vi "Requests.vi"(8 "error in (no error)":errorcluster, 9 "write enable":bool=TRUE, 11 "ICPCON ET-7051 in":refnum<class "ICPCON ET-7051.lvclass">) -> (0 "error out":errorcluster, 3 "ICPCON ET-7051 out":refnum<class "ICPCON ET-7051.lvclass">)   [LabVIEW 2019, in "ICPCON ET-7051.lvclass"]
uses:
  ICPCON ET-7051.lvclass
  D:/my_projects/projects/Algorithms/Labview/19/Modbus/MB_TCP2/MB_TCP.lvclass
  MB_TCP.lvclass/MB_TCP.ctl
  NI_modbus_upd/Ctl/Unit_ID.ctl
  NI_modbus_upd/TCP/TCP.lvclass/TCP.ctl
  NI_modbus_upd/Master Function Definition/Responses/Read Discrete Inputs Response.vi
  NI_modbus_upd/Master network read write.vi
  NI_modbus_upd/Master Function Definition/Requests/Read Discrete Inputs Request.vi
  NI_modbus_upd/Utility/Bytes to Bits1.vi
  NI_modbus_upd/Function code mismatch error1.vi
  NI_modbus_upd/Error Generator1.vi
  NI_modbus_upd/Read ADU Packet Master.vi
  NI_modbus_upd/Write ADU Packet Master.vi
  NI_modbus_upd/Modbus Data Unit (PDU)/Construct PDU1.vi
  NI_modbus_upd/Modbus Data Unit (PDU)/Unflatten to PDU1.vi
  NI_modbus_upd/TCP/Protocol Read.vi
  NI_modbus_upd/TCP/Protocol Write.vi
  <vilib>/Utility/error.llb/Clear Errors.vi
  NI_modbus_upd/Modbus Data Unit (PDU)/Deconstruct PDU1.vi
  NI_modbus_upd/TCP/TCP.lvclass
  ICPCON Registers/ICPCON Registers.lvlib
  MB_TCP.lvclass
  NI_modbus_upd/NI_modbus_upd.lvlib
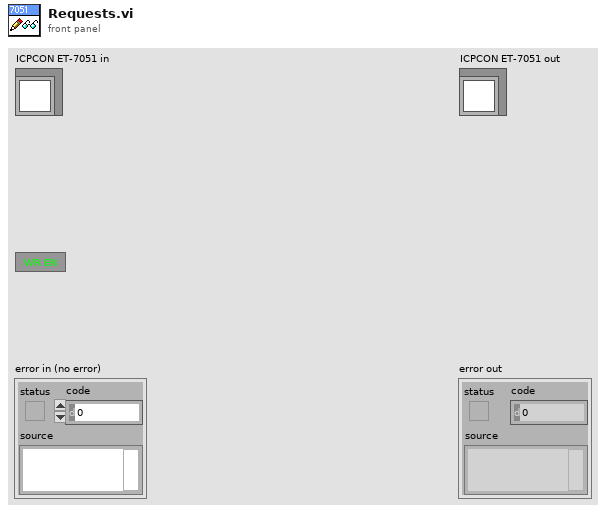
[diagram p1: front panel]
types:
  T1 = typedef "NI_modbus_upd.lvlib/Unit_ID.ctl" = cluster{"Protocol ID":u16, "Unit ID":u8}
  T2 = typedef "ICPCON Registers.lvlib/ICPCON Data.ctl" = cluster{"UTF":refnum<data-value>, "DI":refnum<data-value>, "DW":refnum<data-value>, "DO":refnum<data-value>, "IR":refnum<data-value>, "WR":refnum<data-value>, "OR":refnum<data-value>, "modified":refnum<data-value>}
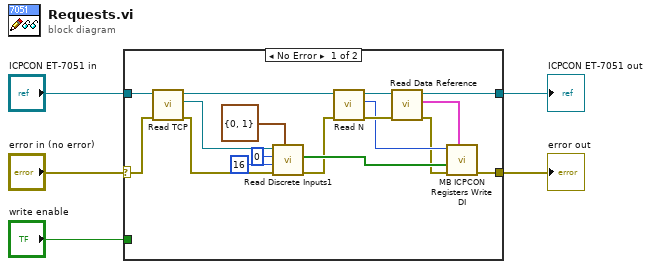
[diagram p0: block diagram]
diagram:
  n1 = case shown="No Error" "error in (no error)" {
    selector: "error in (no error)" -> [w10 w24]
    tunnel: [w16 w24] -> w3
    tunnel: [w9 w23] -> w4
    tunnel: "ICPCON ET-7051 in" -> [w11 w23]
    tunnel: "write enable" -> [_ _]
    frame No Error {
      n2 = call "Read TCP.vi"("error in (no error)"=w10, "MB_TCP in"=w11) -> ("error out"=w19:errorcluster, "TCP"=w20:refnum<class "TCP.lvclass">, "MB_TCP out"=w8:refnum<class "ICPCON ET-7051.lvclass">)  [unwired: 7 in]
      n3 = call "Read Discrete Inputs1.vi"("Unit_ID"=T1 {"Protocol ID"=0, "Unit ID"=1}, "error in (no error)"=w19, "number of discrete inputs"=u16 16, "starting address"=u16 0, "Modbus master in"=w20) -> ("error out"=w6:errorcluster, "discrete input values"=w12:bool[])  [unwired: 4 in, 1 out]
      n4 = call "Read N.vi"("error in (no error)"=w6, "MB_TCP in"=w8) -> ("error out"=w22:errorcluster, "N"=w17:i32, "MB_TCP out"=w21:refnum<class "ICPCON ET-7051.lvclass">)  [unwired: 7 in]
      n5 = call "Read Data Reference.vi"("error in (no error)"=w22, "MB_TCP in"=w21) -> ("error out"=w7:errorcluster, "Data"=w18:T2, "MB_TCP out"=w9:refnum<class "ICPCON ET-7051.lvclass">)  [unwired: 7 in]
      n6 = call "MB ICPCON Registers Write DI.vi"("Data Reference"=w18, "error in (no error)"=w7, "Bits In"=w12, "N"=w17) -> ("error out"=w16:errorcluster)  [unwired: 7 in]
    }
    frame Error {
    }
  }
  "error out" <- w3
  "ICPCON ET-7051 out" <- w4
